vi "ECG_Monitor.vi"() -> ()   [LabVIEW 2026]
uses:
  <vilib>/Analysis/3filter.llb/Filter Passband Type.ctl
  <vilib>/Instr/_visa.llb/VISA Configure Serial Port (Instr).vi
  <vilib>/ptbypt/NI_PtbyPt.lvlib
  <vilib>/Analysis/NI_AALBase.lvlib
panel:
  out "Lie Detector":i32(knob) scale=60.0..90.0
  in  "gain":dbl(slide) scale=0.0..10.0
  out "BPM":dbl
  out "Raw Data":dbl(graph)
  out "Filtered Signal":dbl(graph)
  out "loop iteration":i32
  in  "stop":bool
  out "return count":u32
  out "read buffer":string
  in  "byte count":u32
  in  "Enable Termination\nChar (T)":bool=TRUE
  in  "timeout (10sec)":u32=10000
  in  "termination char\n(0xA = '\\n' = LF)":u8=10 format="%.0x"
  in  "VISA resource name":refnum<visa-resource-name>
  in  "stop bits (10: 1 bit)":u16(ring)=10 items=["1.0"=10, "1.5"=15, "2.0"=20]
  in  "parity (0:none)":enum16{"None", "Odd", "Even", "Mark", "Space"}(ring)
  in  "data bits (8)":u16=8 min=5 max=8 step=1
  in  "baud rate (9600)":u32=9600
  in  "flow control (0:none)":u16(ring) items=["None", "XON/XOFF", "RTS/CTS", "XON/XOFF & RTS/CTS", "DTR/DSR", "XON/XOFF & DTR/DSR"]
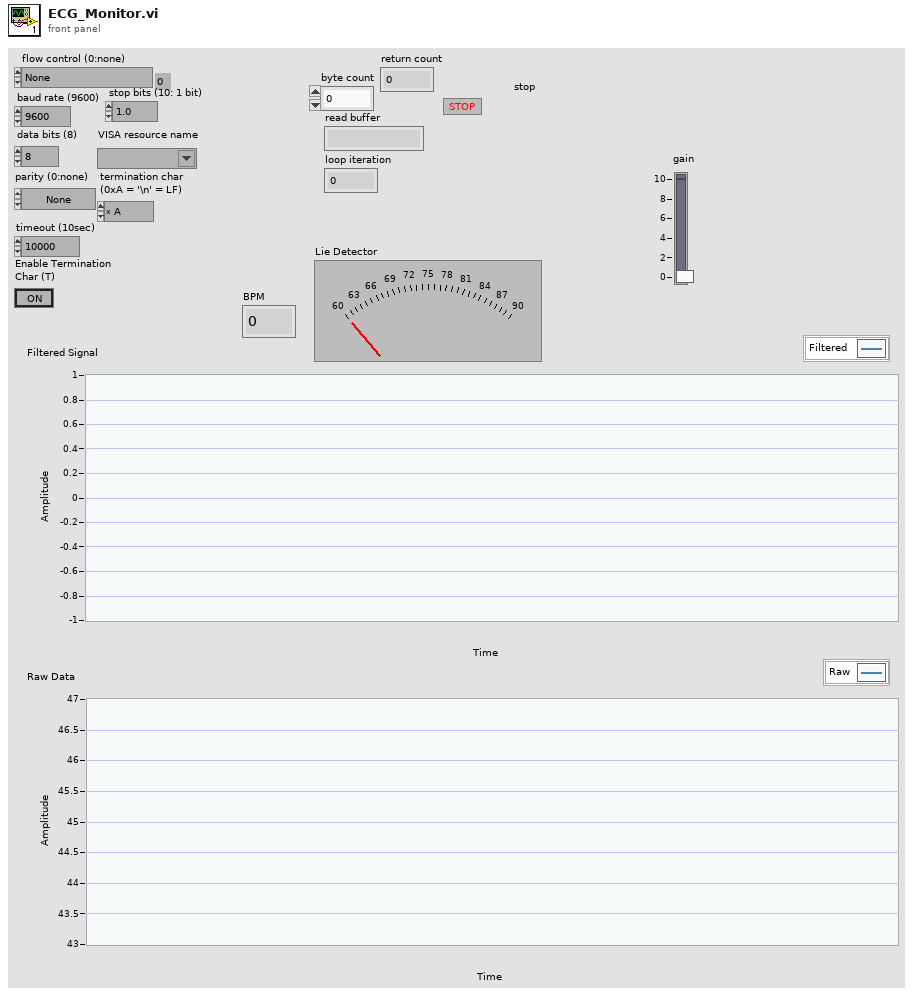
[diagram p1: front panel]
types:
  T1 = typedef "NI_AALBase.lvlib/Filter Passband Type.ctl" = enum32{"Lowpass", "Highpass", "Bandpass", "Bandstop"}
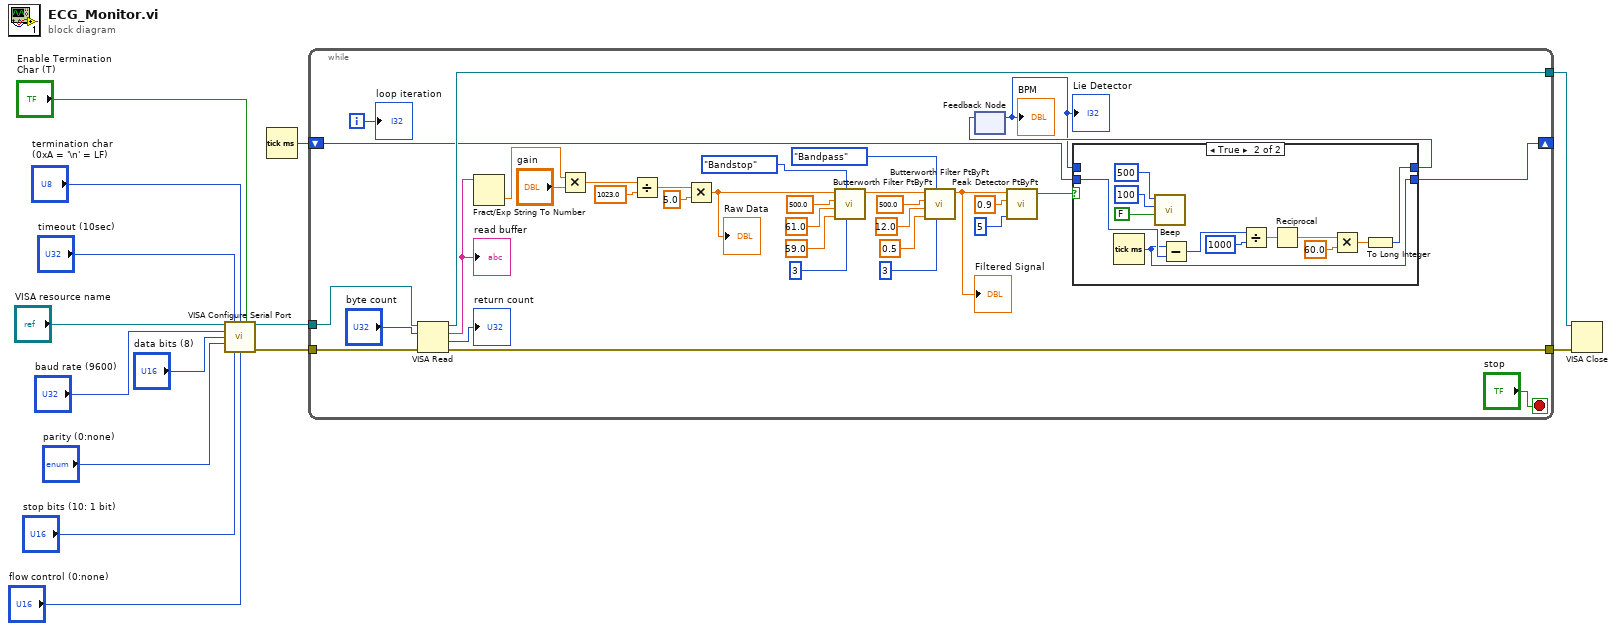
[diagram p0: block diagram]
diagram:
  n1 = call-poly "VISA Configure Serial Port"("VISA resource name"="VISA resource name", "timeout (10sec)"="timeout (10sec)", "termination char\n(0xA = '\\n' = LF)"="termination char\n(0xA = '\\n' = LF)", "Enable Termination\nChar (T)"="Enable Termination\nChar (T)", "baud rate (9600)"="baud rate (9600)", "data bits (8)"="data bits (8)", "parity (0:none)"="parity (0:none)", "stop bits (10: 1 bit)"="stop bits (10: 1 bit)", "flow control (0:none)"="flow control (0:none)") -> ("VISA resource name out"=w5:refnum<visa-resource-name>, "error out"=w4:errorcluster)  [unwired: 5 in]
  n2 = Tick Count (ms)() -> (millisecond timer value=w1:u32)
  n3 = while {
    tunnel: w5 -> [w49]
    tunnel: w4 -> [w48]
    tunnel: [w46] -> w3
    tunnel: [w45] -> w2
    shift-right: [w20] -> _
    shift-left: w1 -> [w21]
    i -> [w30]
    stop <- "stop" stop-if-true
    n4 = VISA Read(VISA resource name=w49, byte count="byte count", error in (no error)=w48) -> (VISA resource name out=w46:refnum<visa-resource-name>, read buffer=w29:string, return count=→"return count":u32, error out=w45:errorcluster)
    "read buffer" <- w29
    n5 = Fract/Exp String To Number(string=w29) -> (number=w18:dbl)  [unwired: 3 in, 1 out]
    n6 = Multiply(x=w18, y="gain") -> (x*y=w17:dbl)
    n7 = Divide(x=w17, y=1023.0) -> (x/y=w42:dbl)
    n8 = Multiply(x=w42, y=5.0) -> (x*y=w28:dbl)
    "Raw Data" <- w28
    n9 = call <vilib>:"Butterworth Filter PtByPt.vi"("order"=3, "filter type"=Filter_Passband_Type."Bandstop", "low cutoff freq: fl"=59.0, "high cutoff freq: fh"=61.0, "sampling freq: fs"=500.0, "x"=w28) -> ("Filtered x"=w40:dbl)  [unwired: 3 in, 1 out]
    n10 = call <vilib>:"Butterworth Filter PtByPt.vi"("order"=3, "filter type"=Filter_Passband_Type."Bandpass", "low cutoff freq: fl"=0.5, "high cutoff freq: fh"=12.0, "sampling freq: fs"=500.0, "x"=w40) -> ("Filtered x"=w26:dbl)  [unwired: 3 in, 1 out]
    "Filtered Signal" <- w26
    n11 = feedback #1() -> (w15:i32)  [unwired: 1 in]
    "BPM" <- w15
    "Lie Detector" <- w15
    n12 = call <vilib>:"Peak Detector PtByPt.vi"("x"=w26, "threshold peak"=0.9, "width"=5) -> ("peak"=w22:bool)  [unwired: 2 in, 2 out]
    n13 = case shown="True" w22 {
      tunnel: w21 -> [w51 w53]
      tunnel: [w51 w52] -> w20
      tunnel: [w50 w54] -> w19
      tunnel: w15 -> [w50 _]
      frame False {
      }
      frame True {
        n14 = Tick Count (ms)() -> (millisecond timer value=w52:u32)
        n15 = call <vilib>:"Beep.vi"("use system alert? (T)"=FALSE, "duration (msec)"=u32 100, "frequency (Hz)"=u32 500) -> ()  [unwired: 9 in]
        n16 = Subtract(x=w52, y=w53) -> (x-y=w60:u32)
        n17 = Divide(x=w60, y=u32 1000) -> (x/y=w58:dbl)
        n18 = Reciprocal(x=w58) -> (1/x=w57:dbl)
        n19 = Multiply(x=w57, y=60.0) -> (x*y=w55:dbl)
        n20 = To Long Integer(number=w55) -> (32bit integer=w54:i32)
      }
    }
    n21 = feedback-in #1(w19) -> ()
    "loop iteration" <- w30
  }
  n22 = VISA Close(VISA resource name=w3, error in (no error)=w2) -> ()  [unwired: 1 out]
